vi "Plotmatrix Max Range.vi"(9 "Current Range Array":T1[][](array[typedef]), 11 "Max Range Array In":T1[][](array[typedef])) -> (3 "Max Range Array Out":T1[][](array[typedef]))   [LabVIEW 2017, in "XY Plot Matrix Datatype.lvclass"]
uses:
  <vilib>/Math Plots/2D Math Plots/XY Plot Matrix/XY Plot Matrix Datatype/XY Plot Matrix Datatype.lvclass
  <vilib>/Math Plots/2D Math Plots/2D Plot/2D Plot/Typedef/Range Cluster.ctl
  <vilib>/Math Plots/2D Math Plots/2D Plot/2D Plot/2D Plot.lvclass
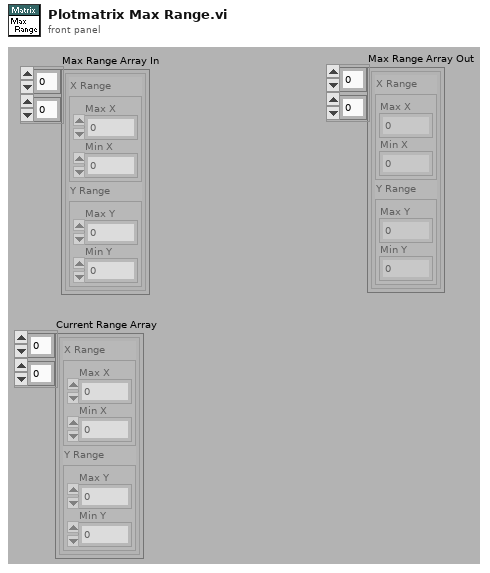
[diagram p1: front panel]
types:
  T1 = typedef "2D Plot.lvclass/Range Cluster.ctl" = cluster{"X Range":cluster{"Max X":dbl, "Min X":dbl}, "Y Range":cluster{"Max Y":dbl, "Min Y":dbl}}
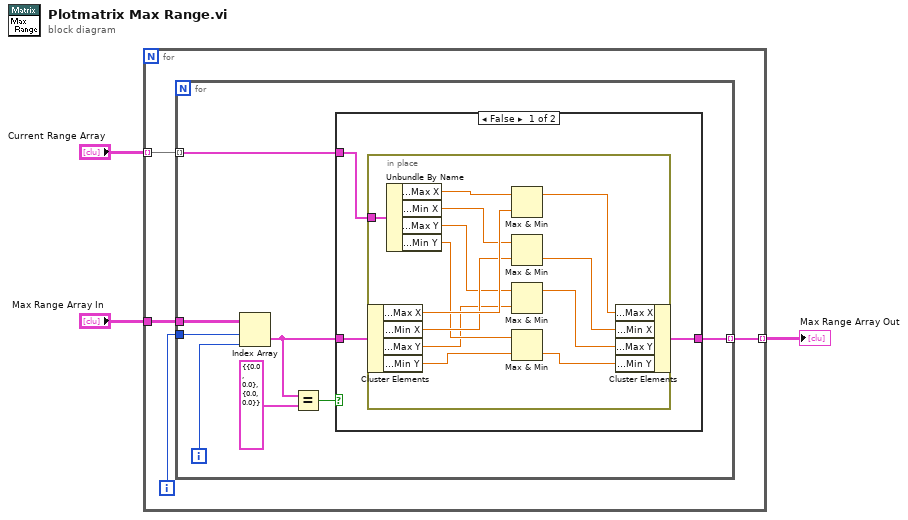
[diagram p0: block diagram]
diagram:
  n1 = for {
    tunnel: "Max Range Array In" -> [w7]
    tunnel: "Current Range Array" -> [w6] mode=indexing
    tunnel: [w5] -> w1 mode=indexing
    i -> [w4]
    n2 = for {
      tunnel: w7 -> [w11]
      tunnel: w6 -> [w13] mode=indexing
      tunnel: [w12] -> w5 mode=indexing
      tunnel: w4 -> [w9]
      i -> [w8]
      n3 = Index Array(array=w11, index (row)=w9, index (col)=w8) -> (element=w10:T1)
      n4 = Equal?(x=w10, y=T1 {"X Range"={"Max X"=0.0, "Min X"=0.0}, "Y Range"={"Max Y"=0.0, "Min Y"=0.0}} ("Max Range In 2")) -> (x = y?=w15:bool)
      n5 = case shown="False" w15 {
        tunnel: w10 -> [w18 _]
        tunnel: w13 -> [w17 w32]
        tunnel: [w16 w32] -> w12
        frame False {
          n6 = in-place {
            in-place-border: w17 -> [w19]
            n7 = in-place-cluster #1(w18) -> ("X Range.Max X"=w30:dbl, "X Range.Min X"=w27:dbl, "Y Range.Max Y"=w21:dbl, "Y Range.Min Y"=w20:dbl)
            n8 = Unbundle By Name(w19) -> ("X Range.Max X"=w31:dbl, "X Range.Min X"=w28:dbl, "Y Range.Max Y"=w22:dbl, "Y Range.Min Y"=w23:dbl)
            n9 = Max & Min(x=w31, y=w30) -> (max(x,y)=w29:dbl)  [unwired: 1 out]
            n10 = Max & Min(x=w28, y=w27) -> (min(x,y)=w26:dbl)  [unwired: 1 out]
            n11 = Max & Min(x=w22, y=w21) -> (max(x,y)=w25:dbl)  [unwired: 1 out]
            n12 = Max & Min(x=w23, y=w20) -> (min(x,y)=w24:dbl)  [unwired: 1 out]
            n13 = in-place-cluster #1("X Range.Max X"=w29, "X Range.Min X"=w26, "Y Range.Max Y"=w25, "Y Range.Min Y"=w24) -> (w16:T1)
          }
        }
        frame True {
        }
      }
    }
  }
  "Max Range Array Out" <- w1
